vi "SetBreakPoints.vi"(5 "Action":u16(ring) items=["No Change", "Reset on Breakpoint", "Set on Breakpoint", "Toggle on Breakpoint"], 6 "error in (no error)":errorcluster, 7 "Step between lines (0)":u32=1000 max=2147483647, 8 "Axis":T4=1 items=["Axis 1"=1, "Axis 2"=2, "Axis 3"=3, "Axis 4"=4, "Axis 5"=5, "Axis 6"=6, "Axis 7"=7, "Axis 8"=8], 9 "Board ID":T3=1 min=1 max=32 step=1) -> (0 "error out":errorcluster, 2 "Program (1) out":T2=1 format="%.0x", 3 "Bd ID Out":T1=1)   [LabVIEW 2022 SP3]
doc: "*NOTE: This example will not work with a FlexMotion-6C. Only one breakpoints is enabled at the beginning of each repeat period. To use modulus breakpoint on a 6C requires waiting until a new repeat period is reached before re-enabling. Please see the online help for \"Load Breakpoint Modulus\" for more information.\n\nDESCRIPTION:\nThe Modulus Breakpoint (on-board re-enable) VI completes a move to a user-specified position on a single axis. During the move, a breakpoint output is asserted an initial user-specified breakpoint position. Relative to the initial breakpoint, more breakpoints will occur at integer multiples of the Breakpoint Modulus. Each time the breakpoint occurs, it must be re-enabled before the next breakpoint modulus is reached. Breakpoint Outputs are commonly used as a digital triggers for another device.\n\nThis example uses an on-board program to re-enable each breakpoint. Using an on-board re-enable will generally respond faster than a host-level re-enable. The breakpoint may set and reset so quickly that the indicator may not detect it, even.\n\nINSTRUCTIONS:\n(1) Be sure your board is initialized before running this VI. Refer to the Initialization topic in the FlexMotion VI Online Help, which can be launched by choosing FlexMotion VI Online Help in the Help menu.\n\n(2) Select the Board ID that corresponds to your FlexMotion controller in the Board Configuration Utility. \n\n(3) Select the axis to be used.\n\n(4) Set the Target Position to which you want the axis to move.\n\n(5) Select the action you want to happen when the breakpoint occurs (set, reset, or toggle).\n\n(6) Set the Breakpoint Position. This is the initial breakpoint position, which must be a value less than the Breakpoint Modulus.\n\n(7) Set the Breakpoint Modulus Position. This is the interval between breakpoints after the initial Breakpoint Position.\n\n(8) Run the VI.\n\nKEY PARAMETERS:\n(1) Target Position: Used to set the position to which the axis should go.\n\n(2) Axis: The number of the axis to be used in the move.\n\n(3) Action: Determines how the breakpoint output will behave when the move crosses the breakpoint position.\n\nI/O CONNECTIONS OVERVIEW:\nThis example requires a system configuration with one axis.\n\n*NOTE: This example is not supported on the 7334 controller."
uses:
  <vilib>/Motion/FlexMotion/CustomControls/CustomControls.llb/Program.flx
  <vilib>/Motion/FlexMotion/FunctionsVIs/OnboardProgramming.llb/Wait on Condition (6 axes).flx
  <vilib>/Motion/FlexMotion/FunctionsVIs/OnboardProgramming.llb/Jump to Label on Condition (6 axes).flx
  <vilib>/Motion/FlexMotion/CustomControls/CustomControls.llb/Axis To Control.flx
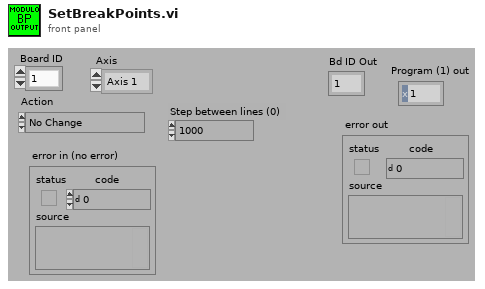
[diagram p1: front panel]
types:
  T1 = typedef "Bd Id Out" = u8
  T2 = typedef "Program.flx" = u8
  T3 = typedef "Board Id" = u8
  T4 = typedef "Axis To Control.flx" = u16
  T5 = enum16{"Reserved0", "Reserved1", "Reserved2", "Reserved3", "Reserved4", "Reserved5", "Reserved6", "Home Found", "Index Found", "High Speed Capture", "Position Breakpoint", "Reserved11", "Velocity Threshold", "Move Complete", "Profile Complete", "Blend Complete", "Motor Off", "Home Input Active", "Limit Input Active", "Software Limit Active", "Program Complete", "IO Port Match"}
  T6 = typedef "Resource Out (Enum).flx" = u16
  T7 = cluster{"0":bool, "1":bool, "2":bool, "3":bool, "4":bool, "5":bool, "6":bool, "7":bool}
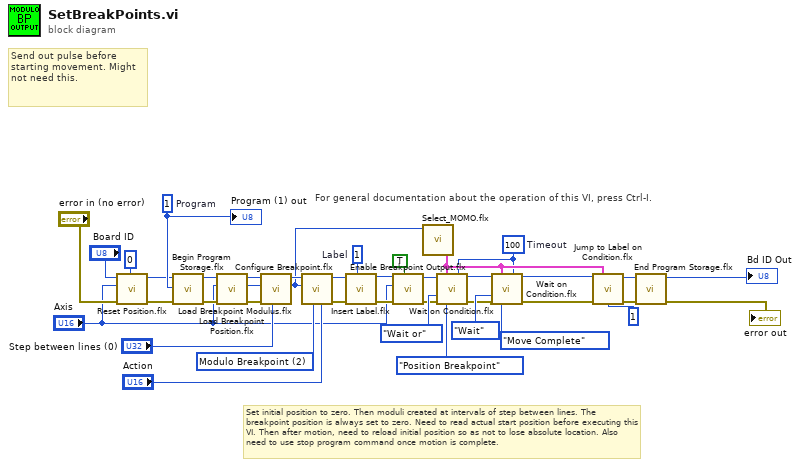
[diagram p0: block diagram]
diagram:
  w21 = u16 2 items=["Absolute Breakpoint", "Relative Breakpoint", "Modulo Breakpoint"] ("Mode")
  w28 = u16 100  # Timeout
  w35 = u16 1  # Label
  w19 = T2 1  # Program
  # "Send out pulse before starting movement. Might not need this."
  # "Set initial position to zero. Then moduli created at intervals of step between lines. The breakpoint position is always set to zero. Need to read actual start position before executing this VI. Then after motion, need to reload initial position so as not to lose absolute location. Also need to use stop program command once motion is complete."
  # "For general documentation about the operation of this VI, press Ctrl-I."
  n1 = call <vilib>:"Reset Position.flx"("Primary Reset Position (0)"=0, "error in (no error)"="error in (no error)", "Axis"="Axis", "Board ID"="Board ID") -> ("error out"=w5:errorcluster, "Bd ID Out"=w6:T1)  [unwired: 1 in, 3 out]
  n2 = call <vilib>:"Begin Program Storage.flx"("error in (no error)"=w5, "Program (1)"=w19, "Board ID"=w6) -> ("error out"=w25:errorcluster, "Bd ID Out"=w36:T1)  [unwired: 4 out]
  n3 = call <vilib>:"Load Breakpoint Position.flx"("error in (no error)"=w25, "Axis or Encoder"="Axis", "Board ID"=w36) -> ("error out"=w38:errorcluster, "Resource Output"=w39:T6, "Bd ID Out"=w40:T1)  [unwired: 1 in, 3 out]
  n4 = call <vilib>:"Load Breakpoint Modulus.flx"("Breakpoint Modulus (0)"="Step between lines (0)", "error in (no error)"=w38, "Axis or Encoder"=w39, "Board ID"=w40) -> ("Resource Output"=w17:T6, "Bd ID Out"=w18:T1)  [unwired: 4 out]
  n5 = call <vilib>:"Configure Breakpoint.flx"("Action (No Change)"="Action", "Mode (Absolute)"=w21, "Axis or Encoder"=w17, "Board ID"=w18) -> ("error out"=w14:errorcluster, "Bd ID Out"=w15:T1)  [unwired: 2 in, 4 out]
  n6 = call <vilib>:"Insert Label.flx"("Label Number (1)"=w35, "error in (no error)"=w14, "Board ID"=w15) -> ("error out"=w13:errorcluster, "Bd ID Out"=w16:T1)  [unwired: 4 out]
  n7 = call <vilib>:"Enable Breakpoint Output.flx"("Enable Breakpoint"=TRUE, "error in (no error)"=w13, "Axis or Encoder"="Axis", "Board ID"=w16) -> ("error out"=w23:errorcluster, "Bd ID Out"=w24:T1)  [unwired: 4 out]
  n8 = call <vilib>:"Select_MOMO.flx"("Resource"=w17) -> ("Must On/Off"=w30:T7)  [unwired: 5 in]
  n9 = call-poly <vilib>:"Wait on Condition.flx"("Board ID"=w24, "Must On"=w30, "Timeout (1)"=w28, "Wait Type (Wait)"=enum16{"Wait", "Wait or"}."Wait or", "error in (no error)"=w23, "Condition Code (Move Complete)"=T5."Position Breakpoint") -> ("Bd ID Out"=w3:T1, "error out"=w4:errorcluster)  [unwired: 3 in, 5 out]
  n10 = call-poly <vilib>:"Wait on Condition.flx"("Board ID"=w3, "Must On"=w30, "Timeout (1)"=w28, "Wait Type (Wait)"=enum16{"Wait", "Wait or"}."Wait", "error in (no error)"=w4, "Condition Code (Move Complete)"=T5."Move Complete") -> ("Bd ID Out"=w2:T1, "error out"=w1:errorcluster)  [unwired: 3 in, 5 out]
  n11 = call-poly <vilib>:"Jump to Label on Condition.flx"("Board ID"=w2, "Must On (False)"=w30, "error in (no error)"=w1, "Jump to Label (1)"=u16 1) -> ("Bd ID Out"=w27:T1, "error out"=w26:errorcluster)  [unwired: 4 in, 6 out]
  n12 = call <vilib>:"End Program Storage.flx"("error in (no error)"=w26, "Board ID"=w27) -> ("error out"=→"error out":errorcluster, "Bd ID Out"=→"Bd ID Out":T1)  [unwired: 1 in, 4 out]
  "Program (1) out" <- w19
